vi "um_to_I32Dim.vi"(6 "-10 to 10V?":bool, 8 "Max Value [um]":dbl, 11 "Input":dbl[](array[numeric])=[0.0, 0.0]) -> (2 "Array":i16[](array[numeric]))   [LabVIEW 2023]
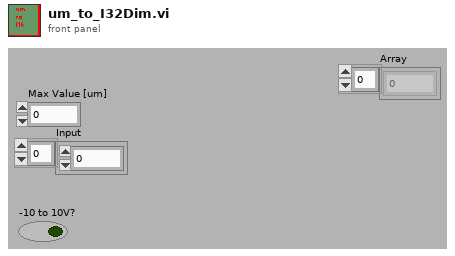
[diagram p1: front panel]
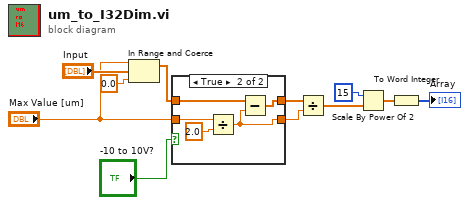
[diagram p0: block diagram]
diagram:
  n1 = In Range and Coerce(upper limit="Max Value [um]", x="Input", lower limit=0.0 ("n")) -> (coerced(x)=w3:dbl[])  [unwired: 1 out]
  n2 = case shown="True" "-10 to 10V?" {
    tunnel: w3 -> [w13 w16]
    tunnel: [w13 w14] -> w5
    tunnel: [w12 w15] -> w4
    tunnel: "Max Value [um]" -> [w12 w17]
    frame False {
    }
    frame True {
      n3 = Divide(x=w17, y=2.0) -> (x/y=w15:dbl)
      n4 = Subtract(x=w16, y=w15) -> (x-y=w14:dbl[])
    }
  }
  n5 = Divide(x=w5, y=w4) -> (x/y=w10:dbl[])
  n6 = Scale By Power Of 2(n=15, x=w10) -> (x*2^n=w9:dbl[])
  n7 = To Word Integer(number=w9) -> (16bit integer=→"Array":i16[])
